vi "parse_create_batch_response.vi"(8 "error_in":errorcluster, 11 "SQL_result":variant) -> (0 "error_out":errorcluster, 2 "batch_ID":string, 3 "batch_code":string)   [LabVIEW 2019]
uses:
  _misc/AULocalize/SubVIs/Get Localized Phrase Compact Interface 0D.vi
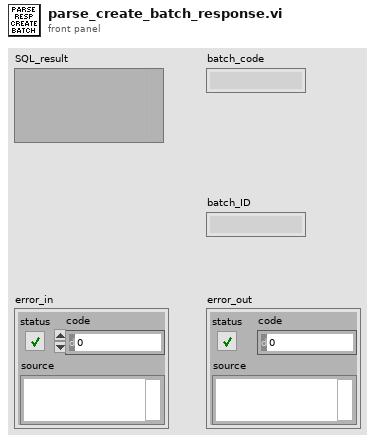
[diagram p1: front panel]
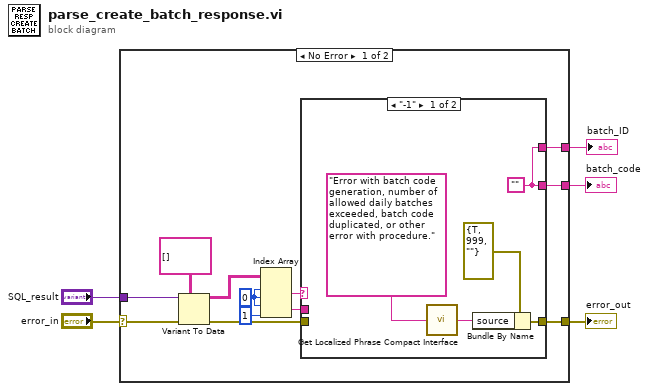
[diagram p0: block diagram]
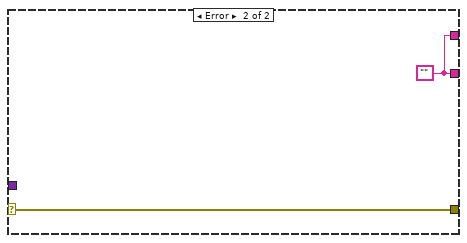
[diagram p3: hidden frame]
diagram:
  n1 = case shown="No Error" "error_in" {
    selector: "error_in" -> [w14 w27]
    tunnel: [w16 w26] -> w5
    tunnel: "SQL_result" -> [w15 _]
    tunnel: [w10 w27] -> w2
    tunnel: [w6 w26] -> w1
    frame No Error {
      w8 = 0 ("disabled index (col)")
      n2 = Variant To Data(error in=w14, type=string[][] [], Variant=w15) -> (data=w12:string[][], error out=w11:errorcluster)
      n3 = Index Array(array=w12, index (row) #1=w8, index (col) #1=w8, index (row) #2=w8, index (col) #2=1 ("disabled index (col)")) -> (element #1=w17:string, element #2=w9:string)
      n4 = case shown="\"-1\"" w17 {
        selector: w17 -> [_ w24]
        tunnel: [w19 w23] -> w16
        tunnel: w11 -> [_ w25]
        tunnel: [w22 w25] -> w10
        tunnel: w9 -> [_ w23]
        tunnel: [w19 w24] -> w6
        frame "-1" {
          w19 = ""
          n5 = call-poly "Get Localized Phrase Compact Interface.vi"("Key"="Error with batch code generation, number of allowed daily batches exceeded, batch code duplicated, or other error with procedure." ("source")) -> ("Translated Phrase"=w18:string)
          n6 = Bundle By Name(cluster=errorcluster {"status"=TRUE, "code"=999, "source"=""} ("error out"), "source"=w18) -> (w22:errorcluster)
        }
        frame Default {
        }
      }
    }
    frame Error {
      w26 = ""
    }
  }
  "error_out" <- w2
  "batch_code" <- w5
  "batch_ID" <- w1
